vi "Set Type.vi"(10 "Type":refnum<class "Type.lvclass">, 11 "TimestampPanel in":refnum<class "TimestampPanel.lvclass">) -> (3 "TimestampPanel out":refnum<class "TimestampPanel.lvclass">)   [LabVIEW 2020, in "Conditum-Tools.lvlib" / "TimestampPanel.lvclass"]
uses:
  TimestampPanel.lvclass
  Conditum-Clone/Columns/Type/Type.lvclass
  TimestampPanel.lvclass/TimestampPanel.ctl
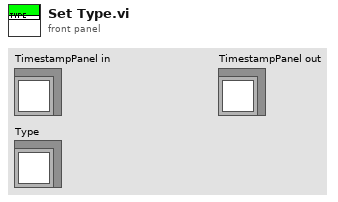
[diagram p1: front panel]
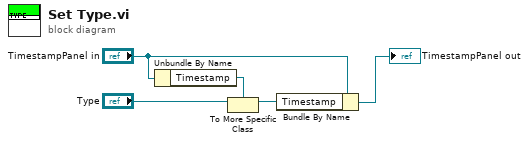
[diagram p0: block diagram]
diagram:
  n1 = Unbundle By Name("TimestampPanel in") -> ("Timestamp"=w4:refnum<class "Timestamp.lvclass">)
  n2 = To More Specific Class(target class=w4, reference="Type") -> (specific class reference=w5:refnum<class "Timestamp.lvclass">)  [unwired: 1 in, 1 out]
  n3 = Bundle By Name(cluster="TimestampPanel in", "Timestamp"=w5) -> (→"TimestampPanel out":refnum<class "TimestampPanel.lvclass">)
